vi "Board Layout Global Variable.vi"() -> ()   [LabVIEW 2016]
panel:
  out "Board Layout":dbl[][](array[numeric])=[[0.0, 2.0, 0.0, 2.0, 0.0, 2.0, 0.0, 2.0], [2.0, 0.0, 2.0, 0.0, 2.0, 0.0, 2.0, 0.0], [0.0, 2.0, 0.0, 2.0, 0.0, 2.0, 0.0, 2.0], [0.0, 0.0, 0.0, 0.0, 0.0, 0.0, 0.0, 0.0], [0.0, 0.0, 0.0, 0.0, 0.0, 0.0, 0.0, 0.0], [1.0, 0.0, 1.0, 0.0, 1.0, 0.0, 1.0, 0.0], [0.0, 1.0, 0.0, 1.0, 0.0, 1.0, 0.0, 1.0], [1.0, 0.0, 1.0, 0.0, 1.0, 0.0, 1.0, 0.0]]
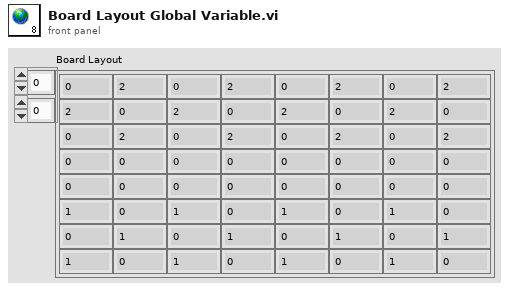
[diagram p1: front panel]
diagram:
